vi "TSM Get Calibration Settings.vi"(0 "TSM context":T2, 11 "error in (no error)":errorcluster) -> (2 "Coarse Freq Sweep (Hz)":T1 {"End" format="%#_13g"; "Start" format="%#_13g"}, 3 "Fine Freq Sweep (Hz)":T1 {"End" format="%#_13g"; "Start" format="%#_13g"}, 4 "TSM context Out":T2, 6 "Coarse Amp Sweep (Hz)":T1 {"End" format="%#_13g"; "Start" format="%#_13g"}, 8 "Fine Amp Sweep (Hz)":T1 {"End" format="%#_13g"; "Start" format="%#_13g"}, 10 "dB SPL Increment":dbl=1.0 format="%#_13g", 13 "Start dB SPL":dbl=60.0 format="%#_13g", 14 "End dB SPL":dbl=130.0 format="%#_13g", 15 "error out":errorcluster)   [LabVIEW 2020]
doc: "Get the DAQmx Analog Output settings of the Speaker from the spec sheet using TSM context"
uses:
  <vilib>/NI_TestStand_SemiconductorModule/NI_TestStand_Semiconductor_Module.lvlibp/PinMap/General/SemiconductorModuleContext.ctl
  Utility/Calibration Sweep/Sweep Parameters.ctl
  <vilib>/NI_TestStand_SemiconductorModule/NI_TestStand_Semiconductor_Module.lvlibp/PinMap/Specs/NamespacedSymbolsToValues.vi
  <vilib>/NI_TestStand_SemiconductorModule/NI_TestStand_Semiconductor_Module.lvlibp
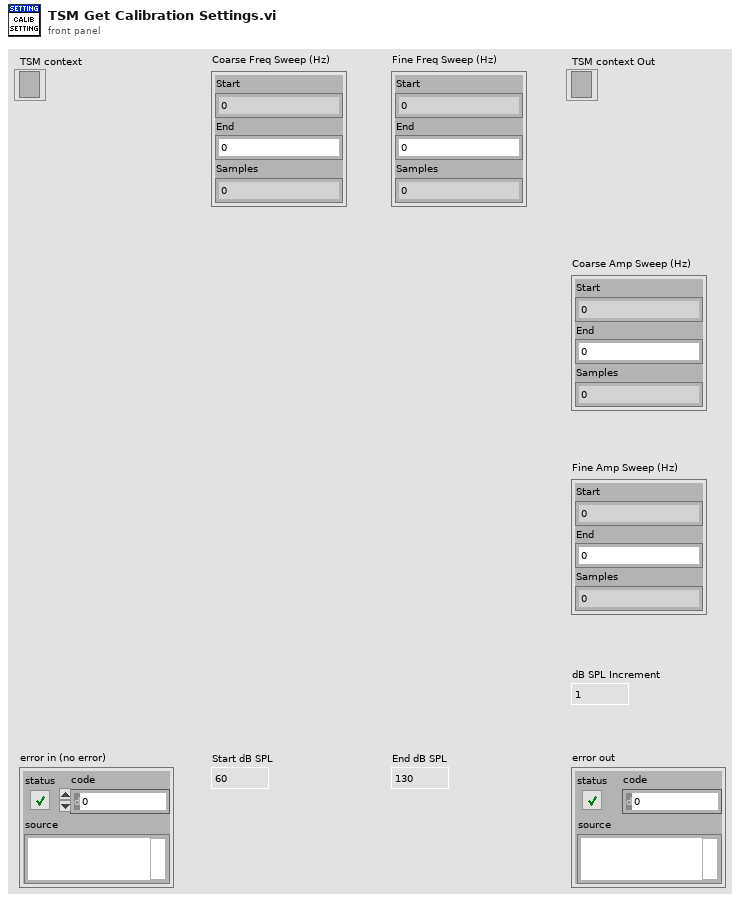
[diagram p1: front panel]
types:
  T1 = typedef "Sweep Parameters.ctl" = cluster{"Start":dbl, "End":dbl, "Samples":i32}
  T2 = typedef "NI_TestStand_Semiconductor_Module.lvlibp/SemiconductorModuleContext.ctl" = refnum<k7>
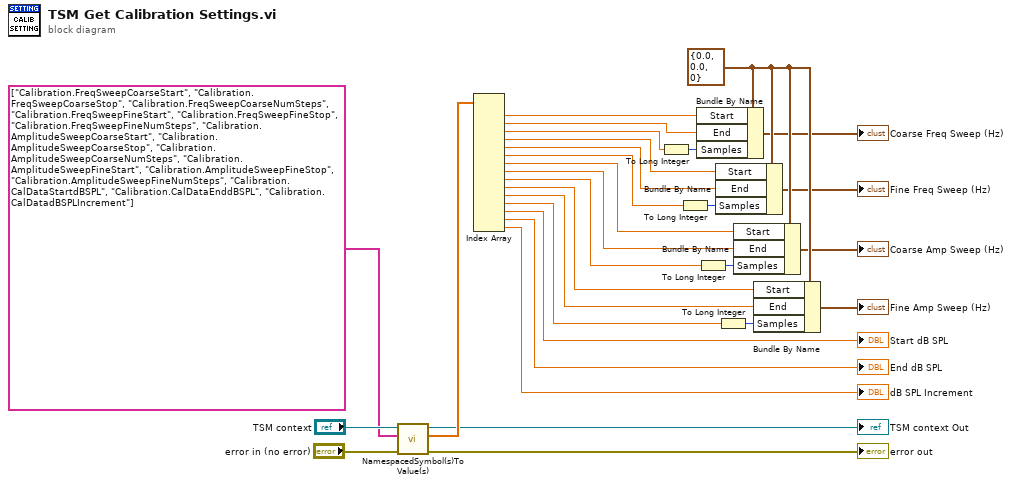
[diagram p0: block diagram]
diagram:
  w8 = T1 {"Start"=0.0, "End"=0.0, "Samples"=0} ("Sweep Parameters")
  n1 = call-poly <vilib>:"NamespacedSymbol(s)ToValue(s).vi"("error in (no error)"="error in (no error)", "Symbols"=tag[] ["Calibration.FreqSweepCoarseStart", "Calibration.FreqSweepCoarseStop", "Calibration.FreqSweepCoarseNumSteps", "Calibration.FreqSweepFineStart", "Calibration.FreqSweepFineStop", "Calibration.FreqSweepFineNumSteps", "Calibration.AmplitudeSweepCoarseStart", "Calibration.AmplitudeSweepCoarseStop", "Calibration.AmplitudeSweepCoarseNumSteps", "Calibration.AmplitudeSweepFineStart", "Calibration.AmplitudeSweepFineStop", "Calibration.AmplitudeSweepFineNumSteps", "Calibration.CalDataStartdBSPL", "Calibration.CalDataEnddBSPL", "Calibration.CalDatadBSPLIncrement"], "Semiconductor Module Context"="TSM context") -> ("error out"=→"error out":errorcluster, "Values"=w27:dbl[], "Semiconductor Module Context Out"=→"TSM context Out":T2)  [unwired: 6 in]
  n2 = Index Array(array=w27) -> (element #1=w24:dbl, element #2=w23:dbl, element #3=w22:dbl, element #4=w19:dbl, element #5=w18:dbl, element #6=w17:dbl, element #7=w14:dbl, element #8=w13:dbl, element #9=w12:dbl, element #10=w11:dbl, element #11=w10:dbl, element #12=w9:dbl, element #13=→"Start dB SPL":dbl, element #14=→"End dB SPL":dbl, element #15=→"dB SPL Increment":dbl)  [unwired: 15 in]
  n3 = To Long Integer(number=w22) -> (32bit integer=w21:i32)
  n4 = To Long Integer(number=w17) -> (32bit integer=w20:i32)
  n5 = Bundle By Name(cluster=w8, "Start"=w24, "End"=w23, "Samples"=w21) -> (→"Coarse Freq Sweep (Hz)":T1)
  n6 = To Long Integer(number=w12) -> (32bit integer=w16:i32)
  n7 = Bundle By Name(cluster=w8, "Start"=w19, "End"=w18, "Samples"=w20) -> (→"Fine Freq Sweep (Hz)":T1)
  n8 = To Long Integer(number=w9) -> (32bit integer=w15:i32)
  n9 = Bundle By Name(cluster=w8, "Start"=w14, "End"=w13, "Samples"=w16) -> (→"Coarse Amp Sweep (Hz)":T1)
  n10 = Bundle By Name(cluster=w8, "Start"=w11, "End"=w10, "Samples"=w15) -> (→"Fine Amp Sweep (Hz)":T1)
